vi "Determine_Meas_Analysis.vi"(1 "Analysis info Cluster In":T1[](array[typedef]) {"Sync Delay Time (s)" format="%.2f"; "Sd Error in Variance" format="%.2f"; "Skew_u" format="%.2f"; "% u'/U" format="%.2f"; "Sd Error in Mean" format="%.2f"; "Kurt_u" format="%.2f"; "u^4" format="%.2f"; "u^3" format="%.2f"; "U" format="%.2f"; "u^2" format="%.2f"}) -> (0 "Analysis info Cluster Out":T1[](array[typedef]) {"Sync Delay Time (s)" format="%.2f"; "Sd Error in Variance" format="%.2f"; "Skew_u" format="%.2f"; "% u'/U" format="%.2f"; "Sd Error in Mean" format="%.2f"; "Kurt_u" format="%.2f"; "u^4" format="%.2f"; "u^3" format="%.2f"; "U" format="%.2f"; "u^2" format="%.2f"})   [LabVIEW 2017]
uses:
  Controls/Analysis_info_cluster.ctl
  Controls/Inst_type.ctl
  Controls/Instrument_Array.ctl
  Globals/Meas_global.vi
  Globals/LDA_meas_global_1.vi
  Globals/LDA_meas_global_2.vi
  Acquisition/PWA/PWAtasksGLOBAL.vi
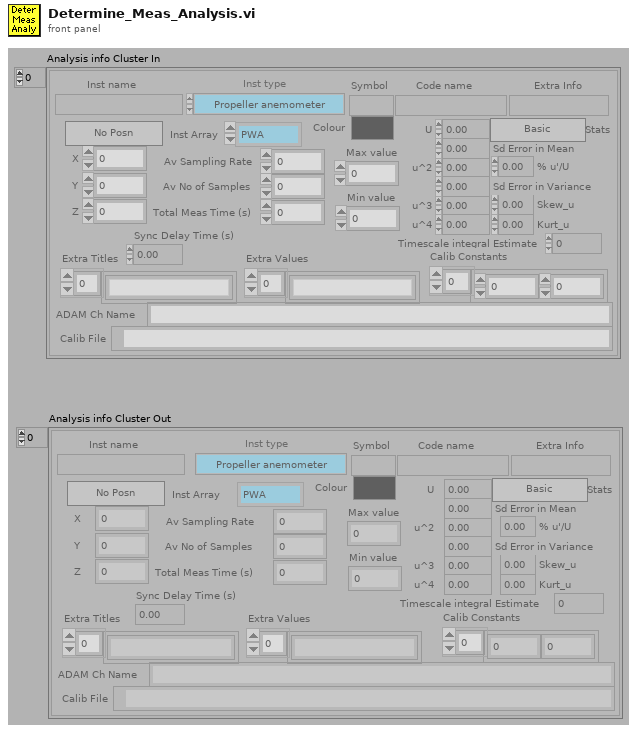
[diagram p1: front panel]
types:
  T1 = typedef "Analysis_info_cluster.ctl" = cluster{"Colour":u32, "Inst type":T2, "Inst name":string, "Symbol":string, "Code name":string, "Extra Info":string, "Inst Array":T3, "Extra Titles":string[], "Extra Values":string[], "U":dbl, "u^2":dbl, "u^3":dbl, "u^4":dbl, "Skew_u":dbl, "Kurt_u":dbl, "Sd Error in Mean":dbl, "% u'/U":dbl, "X":dbl, "Y":dbl, "Z":dbl, "Timescale integral Estimate":dbl, "Sd Error in Variance":dbl, "Calib File":path, "Calib Constants":dbl[], "Output Position":bool, "Full Stats":bool, "Av Sampling Rate":dbl, "Av No of Samples":dbl, "Total Meas Time (s)":dbl, "ADAM Ch Name":string, "Max value":dbl, "Min value":dbl, "Sync Delay Time (s)":dbl}
  T2 = typedef "Inst_type.ctl" = enum16{"Propeller anemometer", "Raw voltage", "Pressure Transducer", "Pitot-static tube", "Preston tube", "Hot wire", "Cross wire 1", "Cross wire 2", "Generic Linear", "Generic Polynomial", "Generic BackPoly", "Fast FID", "Thermocouple", "Cold wire", "Pulsed Wire", "LDA Vel", "LDA Tran time", "LDA Arr time", "Microphone"}
  T3 = typedef "Instrument_Array.ctl" = enum16{"PWA", "LDA", "Analogue"}
  T4 = typedef "BSA_info_Cluster.ctl" = cluster{"GPIB Address":string, "No of Check Bytes":i32, "Extra Info":string, "COLOUR":u32, "Wavelength (nm)":dbl}
  T5 = typedef "LDA_Setup.ctl" = cluster{"dimensions":enum16{"1D", "2D"}, "Analogue Freq Multiplier":dbl}
  T6 = typedef "Post_Process.ctl" = enum16{"Take New Data", "Post Process Raw Data File"}
  T7 = typedef "PWA_Data.ctl" = enum16{"No PWA Data", "One Ch PWA"}
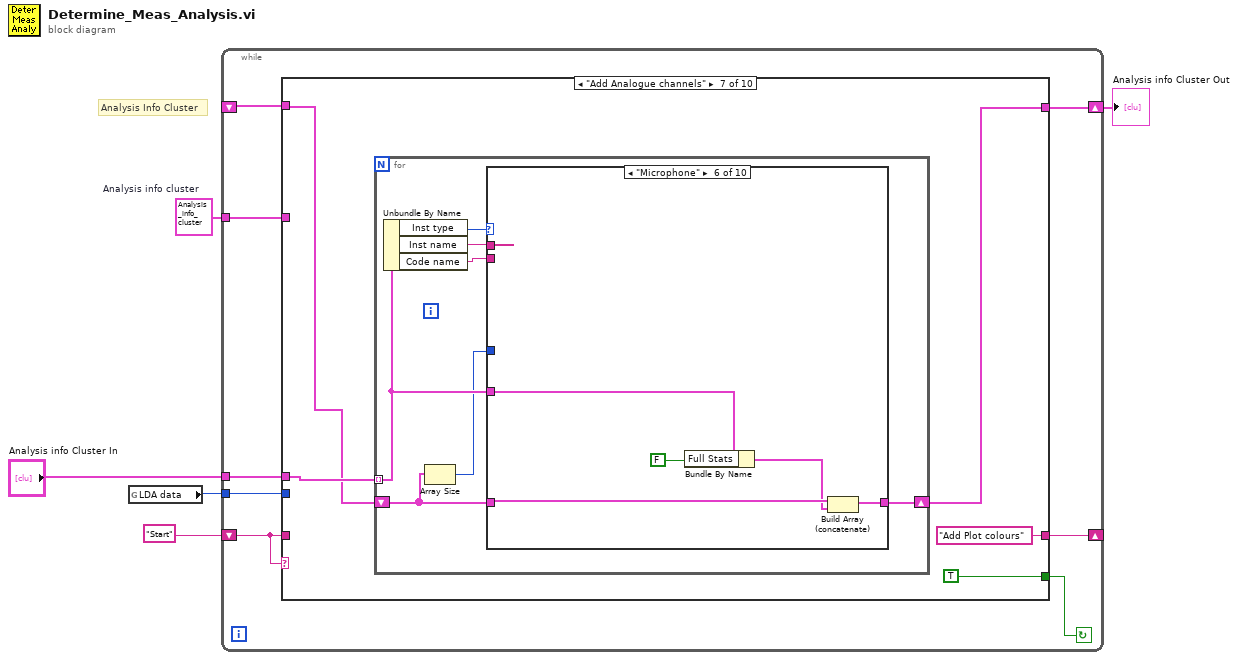
[diagram p0: block diagram]
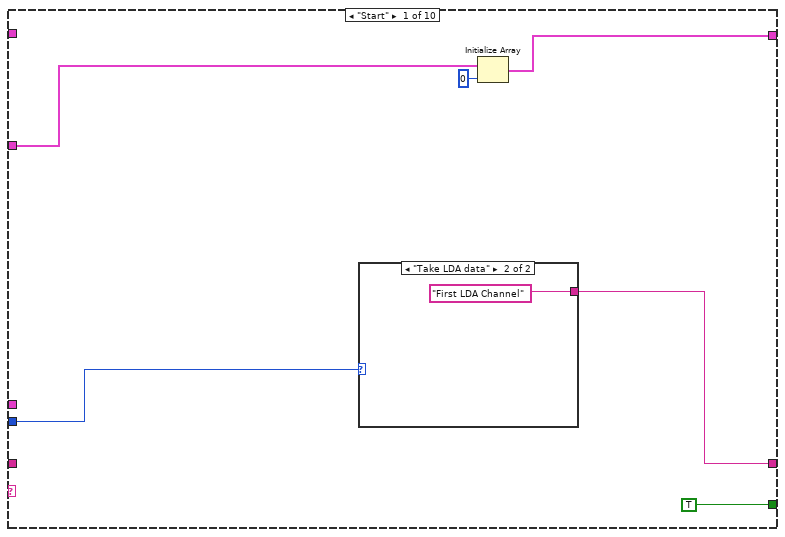
[diagram p2: hidden frame]
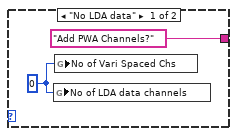
[diagram p3: hidden frame]
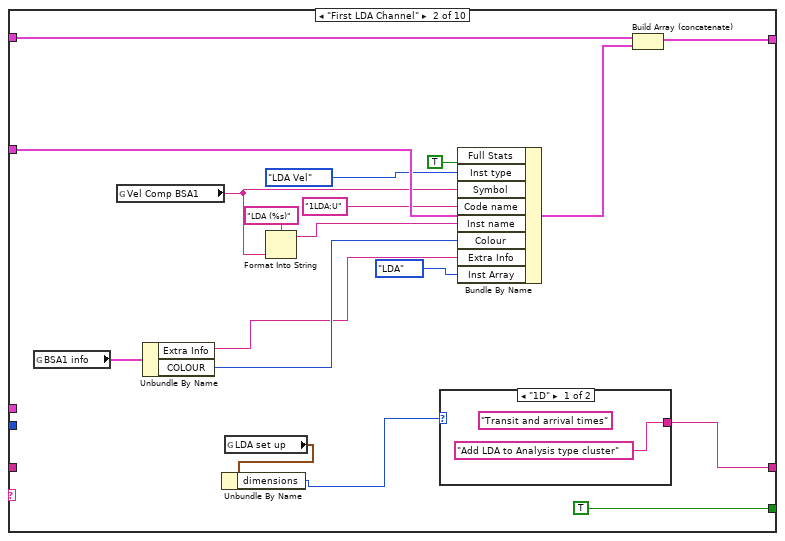
[diagram p4: hidden frame]
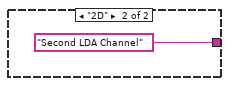
[diagram p5: hidden frame]
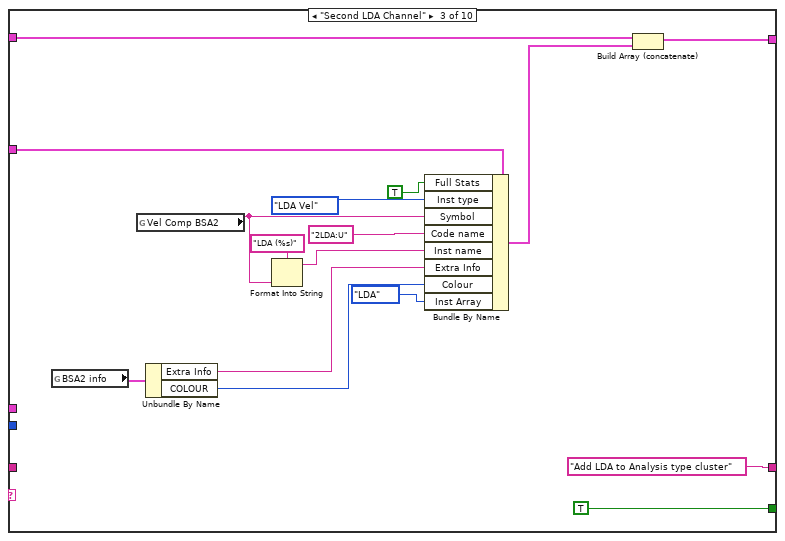
[diagram p6: hidden frame]
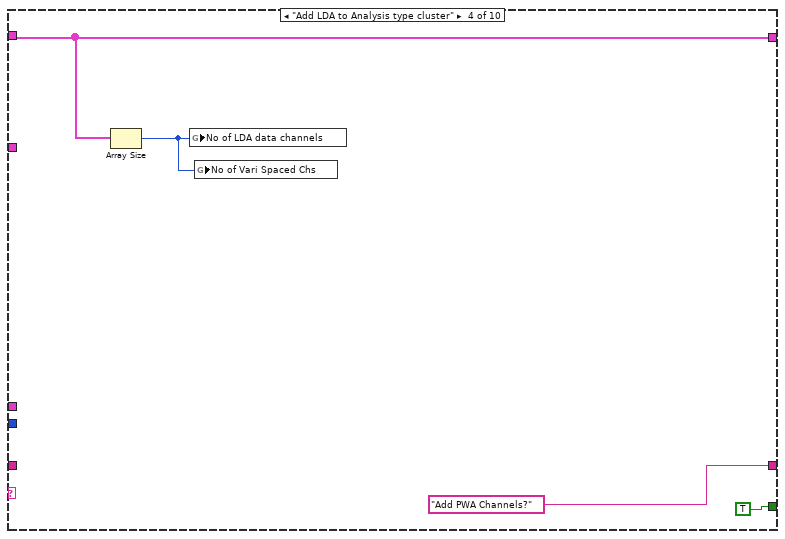
[diagram p7: hidden frame]
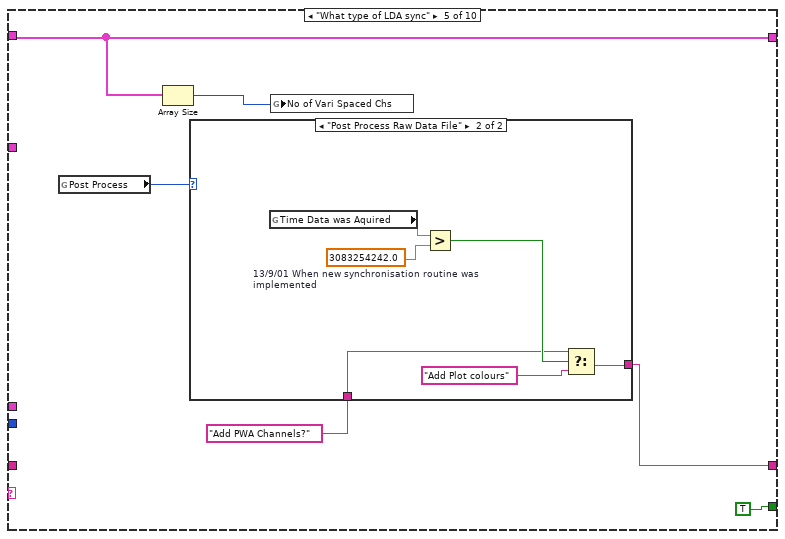
[diagram p8: hidden frame]
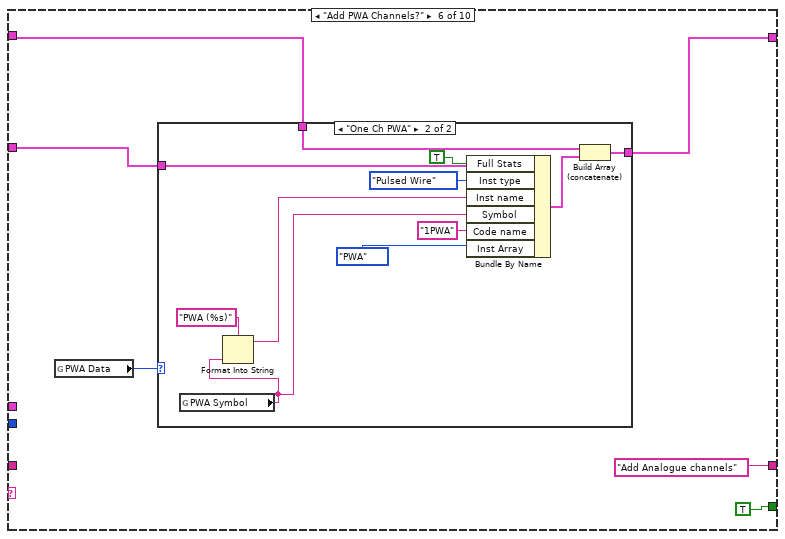
[diagram p10: hidden frame]
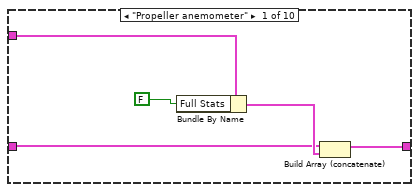
[diagram p12: hidden frame]
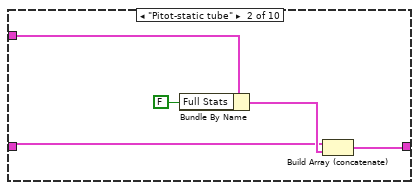
[diagram p13: hidden frame]
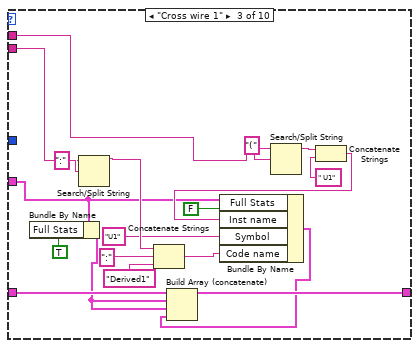
[diagram p14: hidden frame]
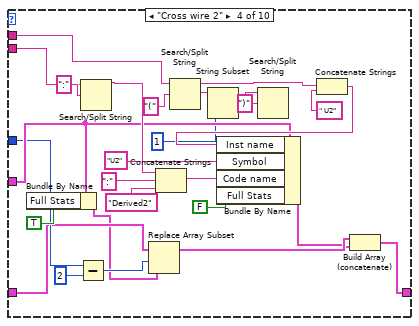
[diagram p15: hidden frame]
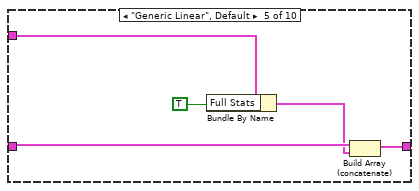
[diagram p16: hidden frame]
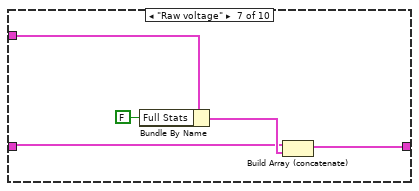
[diagram p17: hidden frame]
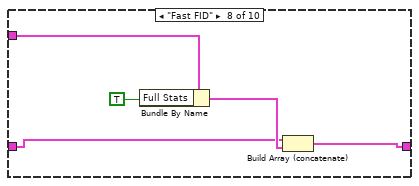
[diagram p18: hidden frame]
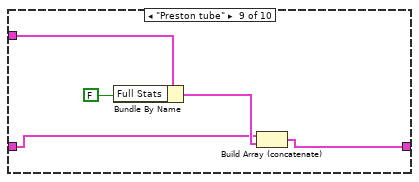
[diagram p19: hidden frame]
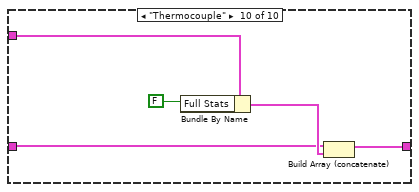
[diagram p20: hidden frame]
diagram:
  w5 = T1 {"Colour"=0, "Inst type"=enum."Pitot-static tube", "Inst name"="Manometer voltage", "Symbol"="U", "Code name"="", "Extra Info"="U", "Inst Array"=enum."PWA", "Extra Titles"=[], "Extra Values"=[], "U"=0.0, "u^2"=0.0, "u^3"=0.0, "u^4"=0.0, "Skew_u"=0.0, "Kurt_u"=0.0, "Sd Error in Mean"=0.0, "% u'/U"=0.0, "X"=0.0, "Y"=0.0, "Z"=0.0, "Timescale integral Estimate"=0.0, "Sd Error in Variance"=0.0, "Calib File"=path "", "Calib Constants"=[], "Output Position"=FALSE, "Full Stats"=FALSE, "Av Sampling Rate"=0.0, "Av No of Samples"=0.0, "Total Meas Time (s)"=0.0, "ADAM Ch Name"="", "Max value"=0.0, "Min value"=0.0, "Sync Delay Time (s)"=0.0}  # Analysis info cluster
  # "Analysis Info Cluster"
  n1 = global read "Meas_global.vi" "LDA data"() -> (w4:enum16{"No LDA data", "Take LDA data"})
  n2 = while {
    tunnel: "Analysis info Cluster In" -> [w8]
    tunnel: w4 -> [w9]
    tunnel: w5 -> [w11]
    shift-left: _ -> [w10]
    shift-right: [w12] -> w2
    shift-right: [w7] -> _
    shift-left: "Start" -> [w6]
    stop <- w13 continue-if-true
    n3 = case shown="\"Add Analogue channels\"" w6 {
      tunnel: [TRUE TRUE TRUE TRUE TRUE TRUE TRUE TRUE FALSE FALSE] -> w13
      tunnel: [w17 w35 w56 w61 w65 w76 w97 w194 w222 w241] -> w12
      tunnel: w11 -> [w16 w39 w55 _ _ w78 _ _ _ _]
      tunnel: w10 -> [_ w37 w57 w61 w65 w77 w94 w195 w222 w241]
      tunnel: w8 -> [_ _ _ _ _ _ w95 _ _ _]
      tunnel: w9 -> [w15 _ _ _ _ _ _ _ _ _]
      tunnel: [w14 w27 "Add LDA to Analysis type cluster" "Add PWA Channels?" w63 "Add Analogue channels" "Add Plot colours" "End" "End" "End"] -> w7
      tunnel: w6 -> [_ _ _ _ _ _ _ _ _ w235]
      frame "Start" {
        n4 = case shown="\"Take LDA data\"" w15 {
          tunnel: ["Add PWA Channels?" "First LDA Channel"] -> w14
          frame "No LDA data" {
            w21 = 0 ("No of LDA data channels")
            n5 = global write "Meas_global.vi" "No of LDA data channels"(w21) -> ()
            n6 = global write "Meas_global.vi" "No of Vari Spaced Chs"(w21) -> ()
          }
          frame "Take LDA data" {
          }
        }
        n7 = Initialize Array(w16, 0 ("Dimension Size")) -> (w17:T1[])
      }
      frame "First LDA Channel" {
        n8 = global read "LDA_meas_global_1.vi" "BSA1 info"() -> (w30:T4)
        n9 = global read "LDA_meas_global_1.vi" "Vel Comp BSA1"() -> (w33:string)
        n10 = Unbundle By Name(w30) -> ("Extra Info"=w28:string, "COLOUR"=w29:u32)
        n11 = global read "Meas_global.vi" "LDA set up"() -> (w24:T5)
        n12 = Unbundle By Name(w24) -> ("dimensions"=w23:enum16{"1D", "2D"})
        n13 = Format Into String(format string="LDA (%s)" ("Format String"), w33) -> (resulting string=w31:string)  [unwired: 2 in, 1 out]
        n14 = case shown="\"1D\"" w23 {
          tunnel: ["Add LDA to Analysis type cluster" "Second LDA Channel"] -> w27
          frame "1D" {
            (unwired) "Transit and arrival times"
          }
          frame "2D" {
          }
        }
        n15 = Bundle By Name(cluster=w39, "Full Stats"=TRUE, "Inst type"=Inst_type."LDA Vel", "Symbol"=w33, "Code name"="1LDA:U" ("Bundle Element"), "Inst name"=w31, "Colour"=w29, "Extra Info"=w28, "Inst Array"=Instrument_Array."LDA" ("Instrument Array")) -> (w36:T1)
        n16 = Build Array (concatenate)(w37, w36) -> (w35:T1[])
      }
      frame "Second LDA Channel" {
        n17 = global read "LDA_meas_global_2.vi" "BSA2 info"() -> (w48:T4)
        n18 = global read "LDA_meas_global_2.vi" "Vel Comp BSA2"() -> (w49:string)
        n19 = Unbundle By Name(w48) -> ("Extra Info"=w46:string, "COLOUR"=w47:u32)
        n20 = Format Into String(format string="LDA (%s)" ("Format String"), w49) -> (resulting string=w51:string)  [unwired: 2 in, 1 out]
        n21 = Bundle By Name(cluster=w55, "Full Stats"=TRUE, "Inst type"=Inst_type."LDA Vel", "Symbol"=w49, "Code name"="2LDA:U" ("Bundle Element"), "Inst name"=w51, "Extra Info"=w46, "Colour"=w47, "Inst Array"=Instrument_Array."LDA" ("Instrument Array")) -> (w50:T1)
        n22 = Build Array (concatenate)(w57, w50) -> (w56:T1[])
      }
      frame "Add LDA to Analysis type cluster" {
        n23 = Array Size(array=w61) -> (size(s)=w60:i32)
        n24 = global write "Meas_global.vi" "No of LDA data channels"(w60) -> ()
        n25 = global write "Meas_global.vi" "No of Vari Spaced Chs"(w60) -> ()
      }
      frame "What type of LDA sync" {
        n26 = global read "Meas_global.vi" "Post Process"() -> (w67:T6)
        n27 = Array Size(array=w65) -> (size(s)=w66:i32)
        n28 = case shown="\"Post Process Raw Data File\"" w67 {
          tunnel: [w69 w71] -> w63
          tunnel: "Add PWA Channels?" -> [w69 w72]
          frame "Take New Data" {
          }
          frame "Post Process Raw Data File" {
            w74 = 3083254242.0  # 13/9/01 When new synchronisation routine was implemented
            n29 = global read "Meas_global.vi" "Time Data was Aquired"() -> (w75:dbl)
            n30 = Greater?(x=w75, y=w74) -> (0:w73:bool)
            n31 = Select(t=w72, s=w73, f="Add Plot colours") -> (s? t:f=w71:string)
          }
        }
        n32 = global write "Meas_global.vi" "No of Vari Spaced Chs"(w66) -> ()
      }
      frame "Add PWA Channels?" {
        n33 = global read "Meas_global.vi" "PWA Data"() -> (w80:T7)
        n34 = case shown="\"One Ch PWA\"" w80 {
          tunnel: w78 -> [_ w93]
          tunnel: w77 -> [w82 w84]
          tunnel: [w82 w91] -> w76
          frame "No PWA Data" {
          }
          frame "One Ch PWA" {
            n35 = global read "PWAtasksGLOBAL.vi" "PWA Symbol"() -> (w85:string)
            n36 = Format Into String(format string="PWA (%s)", w85) -> (resulting string=w86:string)  [unwired: 2 in, 1 out]
            n37 = Bundle By Name(cluster=w93, "Full Stats"=TRUE, "Inst type"=Inst_type."Pulsed Wire", "Inst name"=w86, "Symbol"=w85, "Code name"="1PWA", "Inst Array"=Instrument_Array."PWA") -> (w92:T1)
            n38 = Build Array (concatenate)(w84, w92) -> (w91:T1[])
          }
        }
      }
      frame "Add Analogue channels" {
        n39 = for {
          tunnel: w95 -> [w104] mode=indexing
          shift-right: [w103] -> w97
          shift-left: w94 -> [w100]
          n40 = Unbundle By Name(w104) -> ("Inst type"=w105:T2, "Inst name"=w101:string, "Code name"=w102:string)
          n41 = Array Size(array=w100) -> (size(s)=w99:i32)
          n42 = case shown="\"Microphone\"" w105 {
            tunnel: w101 -> [_ _ w124 w153 _ _ _ _ _ _]
            tunnel: w100 -> [w109 w113 w121 w140 w165 w170 w175 w178 w183 w190]
            tunnel: w104 -> [w107 w112 w120 w151 w166 w171 w173 w180 w185 w188]
            tunnel: [w108 w114 w123 w135 w163 w168 w174 w179 w184 w189] -> w103
            tunnel: w102 -> [_ _ w122 w152 _ _ _ _ _ _]
            tunnel: w99 -> [_ _ _ w142 _ _ _ _ _ _]
            frame "Propeller anemometer" {
              n43 = Bundle By Name(cluster=w107, "Full Stats"=FALSE) -> (w110:T1)
              n44 = Build Array (concatenate)(w109, w110) -> (w108:T1[])
            }
            frame "Pitot-static tube" {
              n45 = Bundle By Name(cluster=w112, "Full Stats"=FALSE) -> (w115:T1)
              n46 = Build Array (concatenate)(w113, w115) -> (w114:T1[])
            }
            frame "Cross wire 1" {
              n47 = Bundle By Name(cluster=w120, "Full Stats"=TRUE) -> (w117:T1)
              n48 = Search/Split String(string=w122, search string/char (-)=":" ("search char (-)")) -> (substring before match=w128:string)  [unwired: 3 out]
              n49 = Concatenate Strings(w128, ":" ("search char (-)"), "Derived1") -> (w129:string)
              n50 = Search/Split String(string=w124, search string/char (-)="(") -> (substring before match=w133:string)  [unwired: 3 out]
              n51 = Concatenate Strings(w133, " U1") -> (w132:string)
              n52 = Bundle By Name(cluster=w120, "Full Stats"=FALSE, "Inst name"=w132, "Symbol"="U1", "Code name"=w129) -> (w116:T1)
              n53 = Build Array (concatenate)(w121, w117, w117, w116) -> (w123:T1[])
            }
            frame "Cross wire 2" {
              n54 = Bundle By Name(cluster=w151, "Full Stats"=TRUE) -> (w138:T1)
              n55 = Subtract(x=w142, y=2) -> (x-y=w139:i32)
              n56 = Search/Split String(string=w152, search string/char (-)=":" ("search char (-)")) -> (substring before match=w157:string)  [unwired: 3 out]
              n57 = Replace Array Subset(array=w140, new element=w138, index=w139) -> (w137:T1[])
              n58 = Concatenate Strings(w157, ":" ("search char (-)"), "Derived2") -> (w158:string)
              n59 = Search/Split String(string=w153, search string/char (-)="(") -> (substring before match=w148:string, match + rest of string=w146:string)  [unwired: 2 out]
              n60 = String Subset(string=w146, offset (0)=1) -> (substring=w145:string)  [unwired: 1 out]
              n61 = Search/Split String(string=w145, search string/char (-)=")") -> ()  [unwired: 4 out]
              n62 = Concatenate Strings(w148, " U2") -> (w161:string)
              n63 = Bundle By Name(cluster=w151, "Inst name"=w161, "Symbol"="U2", "Code name"=w158, "Full Stats"=FALSE) -> (w136:T1)
              n64 = Build Array (concatenate)(w137, w136) -> (w135:T1[])
            }
            frame "Generic Linear", Default {
              n65 = Bundle By Name(cluster=w166, "Full Stats"=TRUE) -> (w164:T1)
              n66 = Build Array (concatenate)(w165, w164) -> (w163:T1[])
            }
            frame "Microphone" {
              n67 = Bundle By Name(cluster=w171, "Full Stats"=FALSE) -> (w169:T1)
              n68 = Build Array (concatenate)(w170, w169) -> (w168:T1[])
            }
            frame "Raw voltage" {
              n69 = Bundle By Name(cluster=w173, "Full Stats"=FALSE) -> (w176:T1)
              n70 = Build Array (concatenate)(w175, w176) -> (w174:T1[])
            }
            frame "Fast FID" {
              n71 = Bundle By Name(cluster=w180, "Full Stats"=TRUE) -> (w181:T1)
              n72 = Build Array (concatenate)(w178, w181) -> (w179:T1[])
            }
            frame "Preston tube" {
              n73 = Bundle By Name(cluster=w185, "Full Stats"=FALSE) -> (w186:T1)
              n74 = Build Array (concatenate)(w183, w186) -> (w184:T1[])
            }
            frame "Thermocouple" {
              n75 = Bundle By Name(cluster=w188, "Full Stats"=FALSE) -> (w191:T1)
              n76 = Build Array (concatenate)(w190, w191) -> (w189:T1[])
            }
          }
        }
      }
      frame "Add Plot colours" {
        n77 = for {
          tunnel: [w198] -> w194 mode=indexing
          tunnel: w195 -> [w196] mode=indexing
          n78 = Unbundle By Name(w196) -> ("Inst type"=w200:T2, "Colour"=w197:u32)
          n79 = case shown="\"Microphone\"" w200 {
            tunnel: [u32 13421772 u32 13421772 u32 13421772 u32 11711154 u32 6710784 u32 13311 u32 16724736 u32 13382400 u32 10040217 u32 16711935 u32 16711935 u32 16711935 u32 65535 u32 16776960 u32 10027263 u32 10027263 w217 u32 65280 u32 65280] -> w199
            tunnel: w197 -> [_ _ _ _ _ _ _ _ _ _ _ _ _ _ _ _ w217 _ _]
            frame "Propeller anemometer" {
            }
            frame "Pressure Transducer" {
            }
            frame "Microphone" {
            }
            frame "Raw voltage" {
            }
            frame "Pitot-static tube" {
            }
            frame "Preston tube" {
            }
            frame "Hot wire" {
            }
            frame "Cross wire 1" {
            }
            frame "Cross wire 2" {
            }
            frame "Generic Linear" {
            }
            frame "Generic Polynomial" {
            }
            frame "Generic BackPoly" {
            }
            frame "Fast FID" {
            }
            frame "Thermocouple" {
            }
            frame "Cold wire" {
            }
            frame "Pulsed Wire" {
            }
            frame "LDA Vel" {
            }
            frame "LDA Tran time" {
            }
            frame "LDA Arr time" {
            }
          }
          n80 = Bundle By Name(cluster=w196, "Colour"=w199) -> (w198:T1)
        }
      }
      frame "End" {
        n81 = for {
          tunnel: w222 -> [w228] mode=indexing
          shift-right: [w225] -> w220
          shift-left: 0 -> [w226]
          n82 = Unbundle By Name(w228) -> ("Inst Array"=w227:T3)
          n83 = case shown="\"Analogue\"" w227 {
            tunnel: w226 -> [w229 w232 w233]
            tunnel: [w230 w231 w233] -> w225
            frame "PWA" {
              n84 = Increment(x=w229) -> (x+1=w230:i32)
            }
            frame "LDA" {
              n85 = Increment(x=w232) -> (x+1=w231:i32)
            }
            frame "Analogue" {
            }
          }
        }
        n86 = global write "Meas_global.vi" "No of Non Analogue Chs"(w220) -> ()
      }
      frame "No Match", Default {
        n87 = Current VI's Path() -> (path=w236:path)
        n88 = Format Into String(format string="The Case\"%s\" was not Matched\nin VI named\n'%s\"" ("Format String"), w235, w236) -> (resulting string=w239:string)  [unwired: 2 in, 1 out]
        n89 = One Button Dialog(message=w239, button name ("OK")="STOP") -> (true=w237:bool)
        n90 = Stop(stop? (T)=w237) -> ()
      }
    }
  }
  "Analysis info Cluster Out" <- w2
